vi "Write Command.vi"(8 "error in (no error)":errorcluster, 10 "Command?":string, 11 "Serial Device in":refnum<class "Serial Device.lvclass">) -> (0 "error out":errorcluster, 3 "Serial Device out":refnum<class "Serial Device.lvclass">)   [LabVIEW 2016, in "Serial Hardware.lvlib" / "Serial Device.lvclass"]
uses:
  Serial Device.lvclass
  Serial Device.lvclass/Serial Device.ctl
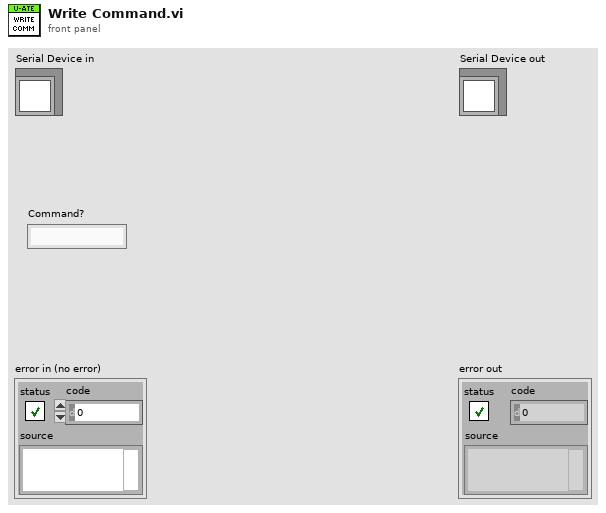
[diagram p1: front panel]
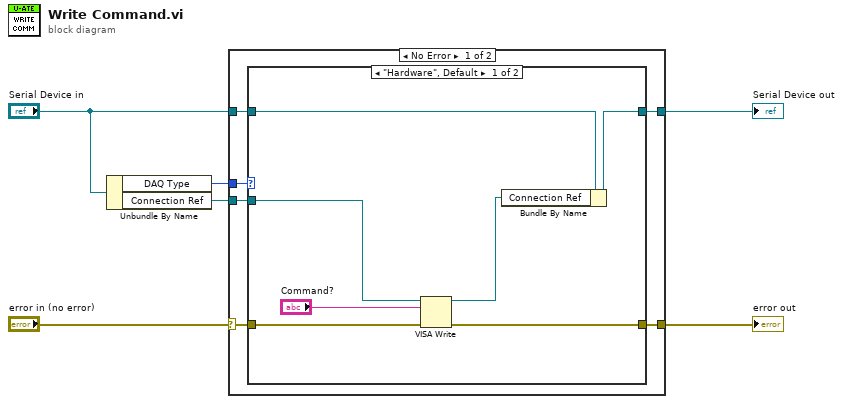
[diagram p0: block diagram]
diagram:
  n1 = Unbundle By Name("Serial Device in") -> ("DAQ Type"=w4:enum16{"Hardware", "Simulation"}, "Connection Ref"=w3:refnum<visa-resource-name>)
  n2 = case shown="No Error" "error in (no error)" {
    selector: "error in (no error)" -> [w8 w22]
    tunnel: "Serial Device in" -> [w10 w23]
    tunnel: w4 -> [w12 _]
    tunnel: w3 -> [w11 _]
    tunnel: [w9 w23] -> w2
    tunnel: [w7 w22] -> w1
    frame No Error {
      n3 = case shown="\"Hardware\", Default" w12 {
        tunnel: w11 -> [w16 _]
        tunnel: w10 -> [w19 w21]
        tunnel: [w14 w21] -> w9
        tunnel: w8 -> [w18 w20]
        tunnel: [w17 w20] -> w7
        frame "Hardware", Default {
          n4 = VISA Write(VISA resource name=w16, write buffer="Command?", error in (no error)=w18) -> (VISA resource name out=w13:refnum<visa-resource-name>, error out=w17:errorcluster)  [unwired: 1 out]
          n5 = Bundle By Name(cluster=w19, "Connection Ref"=w13) -> (w14:refnum<class "Serial Device.lvclass">)
        }
        frame "Simulation" {
        }
      }
    }
    frame Error {
    }
  }
  "error out" <- w1
  "Serial Device out" <- w2
